vi "Trigger_to_IMAQ.vi"() -> ()   [LabVIEW 2015]
panel:
  out "Image":T1(plugin-control)
  in  "Software Trigger":bool
  in  "ICImagingControl":refnum<k7>(container)
  in  "Trigger":bool
  out "Index":i32
  in  "stop":bool
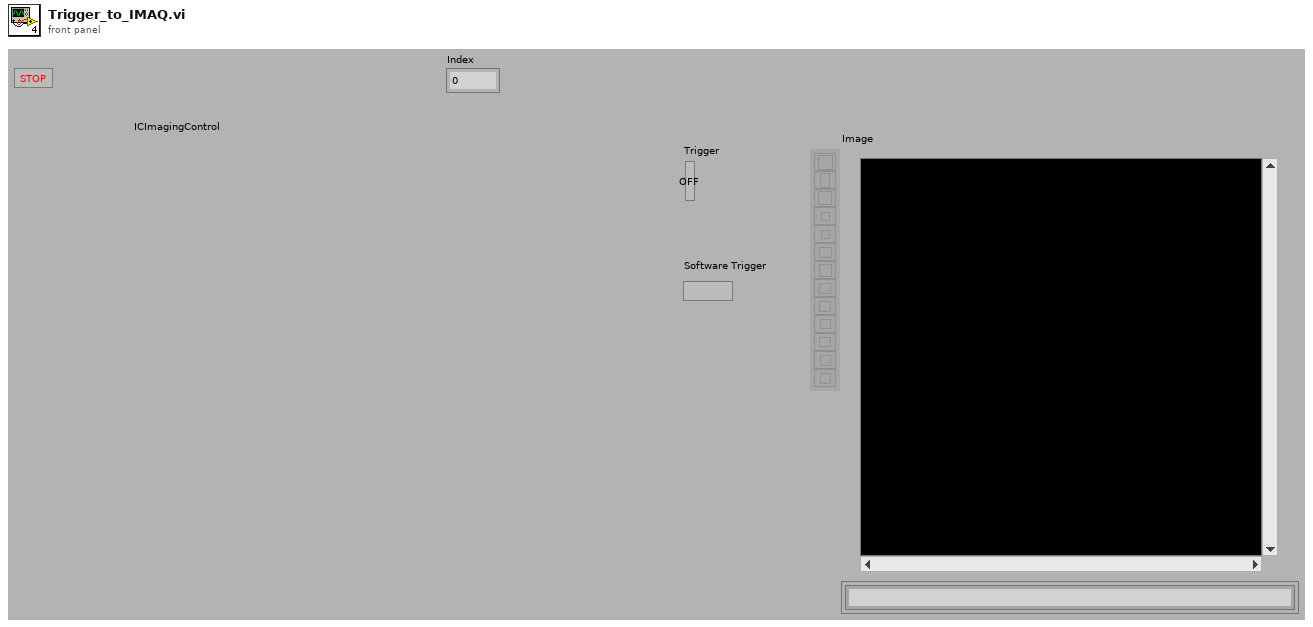
[diagram p1: front panel]
types:
  T1 = typedef "IMAQ Image.ctl" = refnum<image>
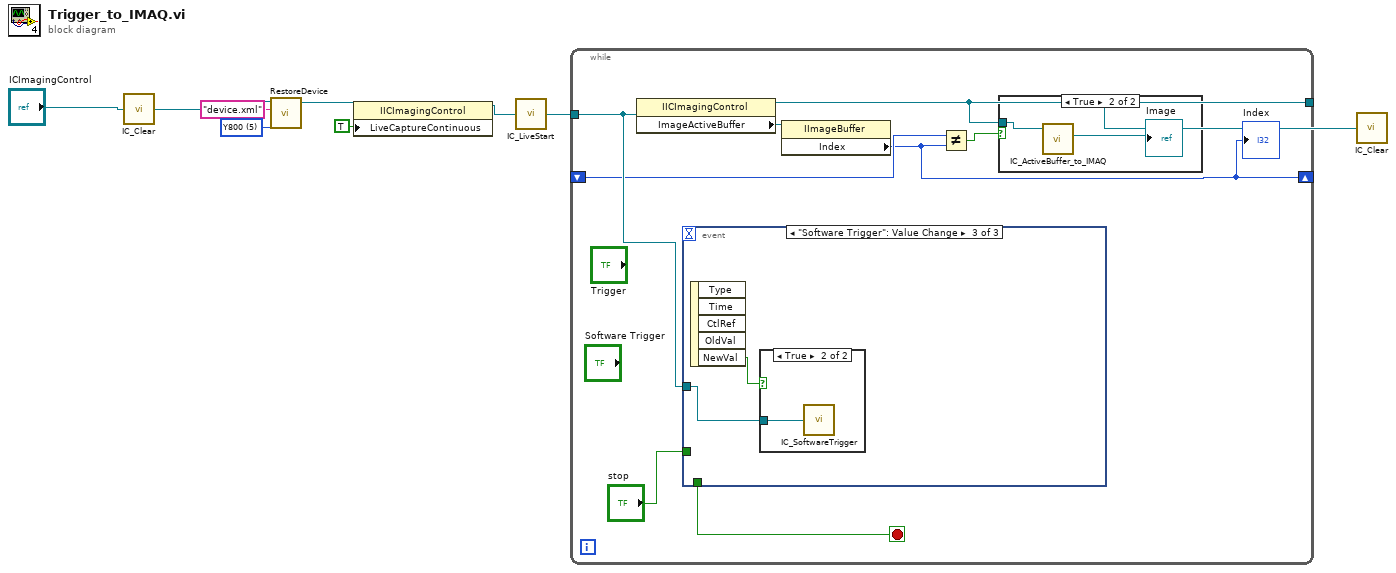
[diagram p0: block diagram]
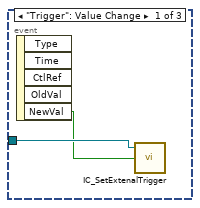
[diagram p3: hidden frame]
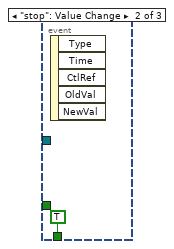
[diagram p4: hidden frame]
diagram:
  w7 = u16 5 items=["RGB"=2, "Y800"=5, "Y16"=11] ("Color modes")
  n1 = call "IC_Clear.vi"("ICImagingControl 2"="ICImagingControl") -> ("ICImagingControl"=w9:refnum<k7>)
  n2 = call "RestoreDevice.vi"("Color modes"=w7, "Filename"="device.xml", "ICImagingControl"=w9) -> ("ICImagingControl 2"=w6:refnum<k7>)  [unwired: 1 in, 2 out]
  n3 = property class="IICImagingControl"(reference=w6, "LiveCaptureContinuous"=TRUE) -> (reference out=w4:refnum<k7>)  [unwired: 1 in, 1 out]
  n4 = call "IC_LiveStart.vi"("ICImagingControl 3"=w4) -> ("ICImagingControl 2"=w3:refnum<k7>)
  n5 = while {
    tunnel: w3 -> [w16]
    tunnel: [w10] -> w2
    shift-right: [w11] -> _
    shift-left: _ -> [w13]
    stop <- w14 stop-if-true
    n6 = property class="IICImagingControl"(reference=w16) -> (reference out=w10:refnum<k7>, "ImageActiveBuffer"=w17:refnum<k7>)  [unwired: 1 in, 1 out]
    n7 = event shown="[2] \"Software Trigger\": Value Change" {
      selector: _ -> [_ _ _]
      dyn-events: _ -> [_ _ _]
      timeout: _ -> [_ _ _]
      tunnel: w16 -> [w21 _ w24]
      tunnel: "stop" -> [_ _ _]
      tunnel: [_ TRUE ("stop") _] -> w14
      event "Trigger": Value Change {
        n8 = event-data() -> ("NewVal"=w20:bool)  [unwired: 1 in, 4 out]
        n9 = call "IC_SetExtenalTrigger.vi"("Trigger"=w20, "ICImagingControl In"=w21) -> ()  [unwired: 1 in, 2 out]
      }
      event "stop": Value Change {
        n10 = event-data() -> ()  [unwired: 1 in, 5 out]
      }
      event "Software Trigger": Value Change {
        n11 = event-data() -> ("NewVal"=w23:bool)  [unwired: 1 in, 4 out]
        n12 = case shown="True" w23 {
          tunnel: w24 -> [_ w25]
          frame False {
          }
          frame True {
            n13 = call "IC_SoftwareTrigger.vi"("ICImagingControl 3"=w25) -> ()  [unwired: 1 out]
          }
        }
      }
    }
    n14 = property class="IImageBuffer"(reference=w17) -> ("Index"=w11:i32)  [unwired: 1 in, 2 out]
    "Index" <- w11
    n15 = Not Equal?(x=w13, y=w11) -> (x != y?=w12:bool)
    n16 = case shown="True" w12 {
      tunnel: w10 -> [_ w19]
      frame False {
      }
      frame True {
        n17 = call "IC_ActiveBuffer_to_IMAQ.vi"("ICImagingControl In"=w19) -> ("Image Out"=→"Image":T1)  [unwired: 2 in, 3 out]
      }
    }
  }
  n18 = call "IC_Clear.vi"("ICImagingControl 2"=w2) -> ()  [unwired: 1 out]
